vi "yokogawa_example.vi"() -> ()   [LabVIEW 2020]
panel:
  in  "Range":T1(ring)
  in  "Current":dbl
  in  "Boolean":bool
  in  "VISA resource name":refnum<visa-resource-name>
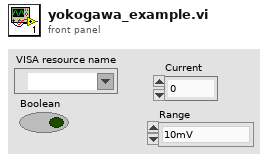
[diagram p1: front panel]
types:
  T1 = enum16{"10mV", "100mV", "1V", "10V", "30V", "1mA", "10mA", "100mA"}
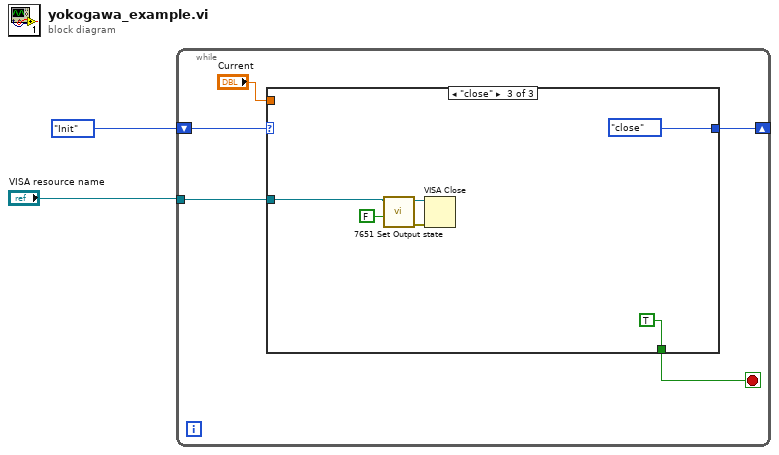
[diagram p0: block diagram]
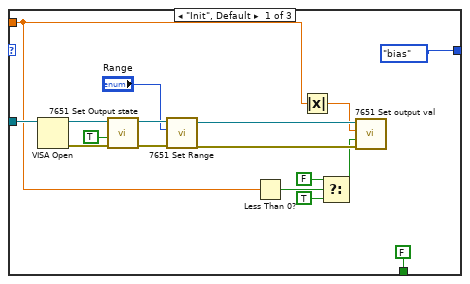
[diagram p2: hidden frame]
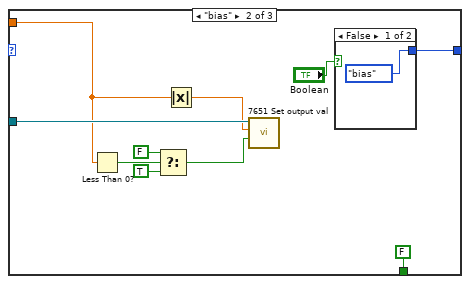
[diagram p3: hidden frame]
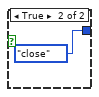
[diagram p4: hidden frame]
diagram:
  n1 = while {
    tunnel: "VISA resource name" -> [w7]
    shift-right: [w6] -> _
    shift-left: enum16{"Init", "bias", "close"}."Init" ("Enum") -> [w3]
    stop <- w5 stop-if-true
    n2 = case shown="\"close\"" w3 {
      tunnel: w7 -> [w17 w33 w37]
      tunnel: [enum16{"Init", "bias", "close"}."bias" ("Enum") w25 enum16{"Init", "bias", "close"}."close" ("Enum")] -> w6
      tunnel: [FALSE FALSE TRUE] -> w5
      tunnel: "Current" -> [w9 w27 _]
      frame "Init", Default {
        n3 = VISA Open(VISA resource name=w17) -> (VISA resource name=w23:refnum<visa-resource-name>, error out=w24:errorcluster)  [unwired: 4 in]
        n4 = call <instrlib>:"7651 Set Output state.vi"("error in"=w24, "Output (F)"=TRUE, "VISA  name"=w23) -> ("error out"=w21:errorcluster, "VISA  name"=w20:refnum<visa-resource-name>)  [unwired: 7 in]
        n5 = call <instrlib>:"7651 Set Range.vi"("error in"=w21, "Range"="Range", "VISA  name"=w20) -> ("error out"=w22:errorcluster, "VISA  name"=w19:refnum<visa-resource-name>)  [unwired: 7 in]
        n6 = Less Than 0?(x=w9) -> (x < 0?=w14:bool)
        n7 = Absolute Value(x=w9) -> (abs(x)=w10:dbl)
        n8 = Select(t=FALSE, s=w14, f=TRUE) -> (s? t:f=w11:bool)
        n9 = call <instrlib>:"7651 Set output val.vi"("error in"=w22, "Pol (T)"=w11, "Val mV/mA (0)"=w10, "VISA  name"=w19) -> ()  [unwired: 6 in, 2 out]
      }
      frame "bias" {
        n10 = Less Than 0?(x=w27) -> (x < 0?=w32:bool)
        n11 = Select(t=FALSE, s=w32, f=TRUE) -> (s? t:f=w29:bool)
        n12 = Absolute Value(x=w27) -> (abs(x)=w28:dbl)
        n13 = call <instrlib>:"7651 Set output val.vi"("Pol (T)"=w29, "Val mV/mA (0)"=w28, "VISA  name"=w33) -> ()  [unwired: 7 in, 2 out]
        n14 = case shown="False" "Boolean" {
          tunnel: [enum16{"Init", "bias", "close"}."bias" ("Enum") enum16{"Init", "bias", "close"}."close" ("Enum")] -> w25
          frame False {
          }
          frame True {
          }
        }
      }
      frame "close" {
        n15 = call <instrlib>:"7651 Set Output state.vi"("Output (F)"=FALSE, "VISA  name"=w37) -> ("error out"=w40:errorcluster, "VISA  name"=w39:refnum<visa-resource-name>)  [unwired: 8 in]
        n16 = VISA Close(VISA resource name=w39, error in (no error)=w40) -> ()  [unwired: 1 out]
      }
    }
  }
